vi "MDAQ_LS335.vi"() -> ()   [LabVIEW 2021]
panel:
  in  "TempB":dbl
  in  "TempA":dbl
  out "Connected":bool
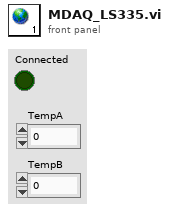
[diagram p1: front panel]
diagram:
